vi "Pre Test Messdaten sammeln.vi"(11 "error in (no error)":errorcluster caption="Fehler (Eingang, kein Fehler)") -> (4 "Messdaten":sgl, 15 "error out":errorcluster caption="Fehler (Ausgang)")   [LabVIEW 2020, in "EPA 1065.lvlib" / "Pre-test verification 1065-520.lvlib"]
uses:
  Pre-test verification 1065-520.lvlib
  Messdaten/Aktionen FGV Messdaten.ctl
  Seiten/FT-IR/Aktionen EVID-Codes.ctl
  Seiten/FT-IR/FGV FT-IR Aktionen.ctl
  Messdaten/Gewichtung (Stichprobe).ctl
  Seiten/FT-IR/FGV FT-IR Gasliste Aktionen.ctl
  Messdaten/Messdaten.lvlib
  Seiten/FT-IR/FT-IR.lvlib
  Allgemein/allgemeine Sub-VIs.lvlib
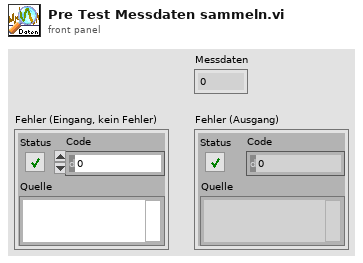
[diagram p1: front panel]
types:
  T1 = typedef "FT-IR.lvlib/FGV FT-IR Gasliste Aktionen.ctl" = enum16{"lesen", "Gasliste FT-IR", "Gasliste ausgelesen", "laden", "speichern", "löschen"}
  T2 = typedef "Messdaten.lvlib/Gewichtung (Stichprobe).ctl" = enum16{"Sample", "Population"}
  T3 = typedef "FT-IR.lvlib/FGV FT-IR Aktionen.ctl" = enum16{"lesen", "NOG setzen", "NOS setzen", "Initialisieren", "speichern", "ALLES setzen", "FT-IR Spektrum loggen", "Komm Stoppen", "Spektrum LogKonfig"}
  T4 = typedef "FT-IR.lvlib/Aktionen EVID-Codes.ctl" = enum16{"lesen", "setzen", "laden", "speichern", "1Hz/5Hz", "Smoothing", "Rolling Average"}
  T5 = typedef "Messdaten.lvlib/Aktionen FGV Messdaten.ctl" = enum16{"lesen", "schreiben", "löschen", "Mittelwerte", "Komponente"}
  T6 = typedef "FT-IR.lvlib/1Hz-5Hz Geraet.ctl" = u16
  T7 = typedef "String - Ausgabefeld.ctl" = string
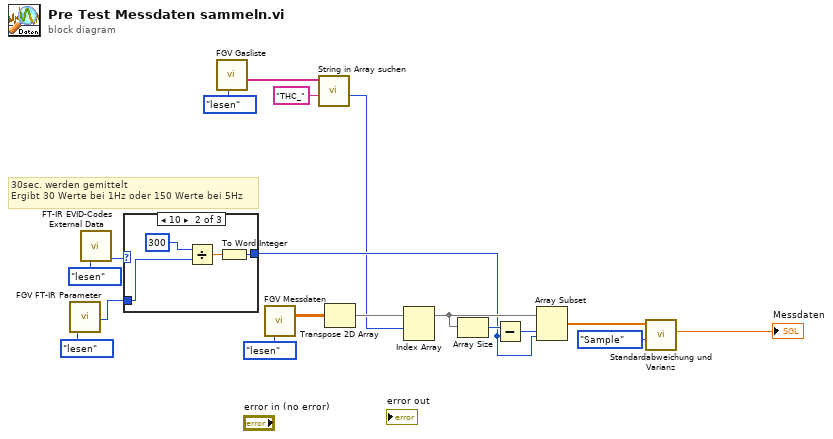
[diagram p0: block diagram]
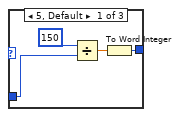
[diagram p2: hidden frame]
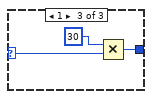
[diagram p3: hidden frame]
diagram:
  # "30sec. werden gemittelt\nErgibt 30 Werte bei 1Hz oder 150 Werte bei 5Hz"
  n1 = call "FGV FT-IR Parameter.vi"("Aktion"=FGV_FT-IR_Aktionen."lesen") -> ("NoOfScan"=w13:u32)  [unwired: 11 in, 7 out]
  n2 = call "FT-IR EVID-Codes External Data.vi"("Aktionen"=Aktionen_EVID-Codes."lesen") -> ("1Hz/5Hz Gerät"=w14:T6)  [unwired: 9 in, 5 out]
  n3 = case shown="10" w14 {
    selector: w14 -> [_ _ w27]
    tunnel: [w19 w23 w28] -> w6
    tunnel: w13 -> [w21 w25 _]
    frame 5, Default {
      n4 = Divide(x=150, y=w21) -> (x/y=w20:dbl)
      n5 = To Word Integer(number=w20) -> (16bit integer=w19:i16)
    }
    frame 10 {
      n6 = Divide(x=300, y=w25) -> (x/y=w24:dbl)
      n7 = To Word Integer(number=w24) -> (16bit integer=w23:i16)
    }
    frame 1 {
      n8 = Multiply(x=30, y=w27) -> (x*y=w28:i32)
    }
  }
  n9 = call "FGV Gasliste.vi"("Aktionen"=FGV_FT-IR_Gasliste_Aktionen."lesen") -> ("Aktuelle Gasliste gesamt"=w2:T7[])  [unwired: 8 in, 2 out]
  n10 = call "FGV Messdaten.vi"("Aktionen"=Aktionen_FGV_Messdaten."lesen") -> ("Messdaten"=w17:sgl[][])  [unwired: 6 in, 8 out]
  n11 = call "String in Array suchen.vi"("Nach String/Zeichen suchen (-)"="THC_", "String-Array"=w2) -> ("Index"=w1:i32)  [unwired: 7 in, 2 out]
  n12 = Transpose 2D Array(2D array=w17) -> (transposed array=w12:sgl[][])
  n13 = Index Array(array=w12, index (row)=w1) -> (element=w8:sgl[])  [unwired: 1 in]
  n14 = Array Size(array=w8) -> (size(s)=w11:i32)
  n15 = Subtract(x=w11, y=w6) -> (x-y=w7:i32)
  n16 = Array Subset(array=w8, index=w7, length=w6) -> (w9:sgl[])
  n17 = call "Standardabweichung und Varianz.vi"("Gewichtung (Stichprobe)"=Gewichtung_(Stichprobe)."Sample", "X"=w9) -> ("Mittelwert"=→"Messdaten":sgl)  [unwired: 7 in, 2 out]
